vi "Create Property.vi"(8 "error in":errorcluster, 10 "Labview Type":T1, 11 "Description":string) -> (0 "error out":errorcluster, 3 "JSON Schema Property out":string)   [LabVIEW 2020, in "JSON Schema Generator.lvlib"]
uses:
  JSON Schema Generator.lvlib
  <vilib>/Utility/Data Type/Type Definitions/Data Type.ctl
  d44ae6e5-6ab7-4cb2-bc4b-87ef910da0f9.vi
  aea4ecb6-ee08-4fcf-bd9c-6a72ca557f06.vi
  <vilib>/JDP Science/JSONtext/Variant to JSON Text.vi
  <vilib>/JDP Science/JSONtext/LVClass Serializer/JSONtext LVClass Serializer.lvclass
  <vilib>/JDP Science/JSONtext/JSONtext.lvlib
  <vilib>/Utility/Data Type/NI_Data Type.lvlib
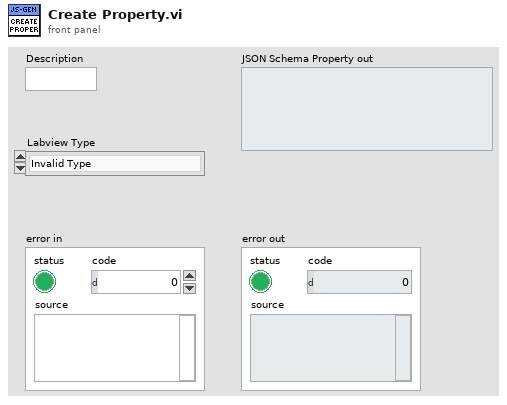
[diagram p1: front panel]
types:
  T1 = typedef "NI_Data Type.lvlib/Data Type.ctl" = enum8{"Invalid Type", "Void", "I8", "I16", "I32", "I64", "U8", "U16", "U32", "U64", "Single Float", "Double Float", "Extended Float", "Single Complex", "Double Complex", "Extended Complex", "Enum U8", "Enum U16", "Enum U32", "Enum U64", "Single Float With Unit", "Double Float With Unit", "Extended Float With Unit", "Single Complex with Unit", "Double Complex with Unit", "Extended Complex with Unit", "Boolean", "String", "Path", "Picture", "Tag", "Array", "Cluster", "Variant", "LV Variant", "Waveform", "Timestamp", "Digital Waveform", "Digital Data", "ExpressData", "Refnum", "External Data", "VI", "Poly VI", "LabVIEW Class Instance", "Fixed Point", "Set Collection", "Map Collection"}
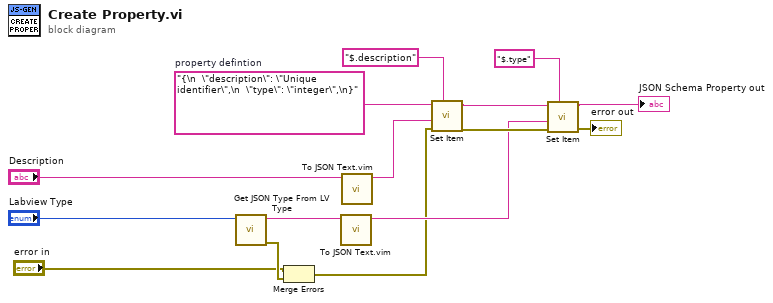
[diagram p0: block diagram]
diagram:
  w12 = "{\n  \"description\": \"Unique identifier\",\n  \"type\": \"integer\",\n}"  # property defintion
  n1 = call "Get JSON Type From LV Type.vi"("Labview Datatype"="Labview Type") -> ("error out"=w14:errorcluster, "JSON Schema Type"=w4:string)  [unwired: 9 in]
  n2 = Merge Errors("error in", w14) -> (w2:errorcluster)
  n3 = call "To JSON Text.vim"("Anything"=w4) -> ("<JSON>"=w7:string)  [unwired: 9 in, 1 out]
  n4 = call "To JSON Text.vim"("Anything"="Description") -> ("<JSON>"=w8:string)  [unwired: 9 in, 1 out]
  n5 = call <vilib>:"Set Item.vi"("$Path or Item Name"="$.description", "error in (no error)"=w2, "JSON to Insert"=w8, "JSON"=w12) -> ("error out"=w13:errorcluster, "<JSON>"=w9:string)  [unwired: 4 in, 1 out]
  n6 = call <vilib>:"Set Item.vi"("$Path or Item Name"="$.type", "error in (no error)"=w13, "JSON to Insert"=w7, "JSON"=w9) -> ("error out"=→"error out":errorcluster, "<JSON>"=→"JSON Schema Property out":string)  [unwired: 4 in, 1 out]
